vi "guerra.vi"(8 "carri difesa":i32, 11 "carri attacco":i32) -> (0 "difesa perde":bool, 2 "carri attacco\nrimanenti":i32, 3 "attacco perde":bool)   [LabVIEW 2013]
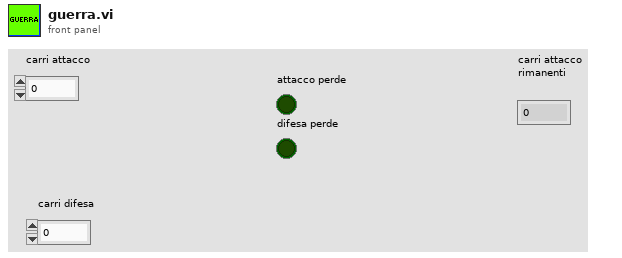
[diagram p1: front panel]
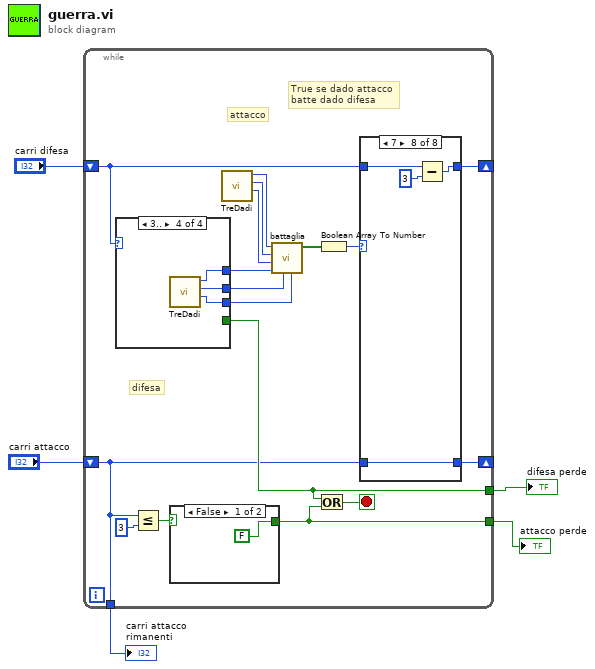
[diagram p0: block diagram]
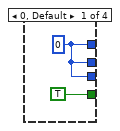
[diagram p2: hidden frame]
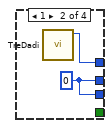
[diagram p3: hidden frame]
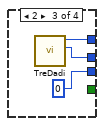
[diagram p4: hidden frame]
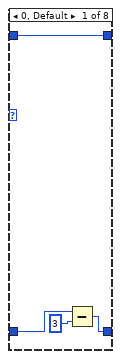
[diagram p5: hidden frame]
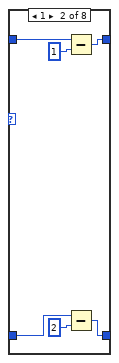
[diagram p6: hidden frame]
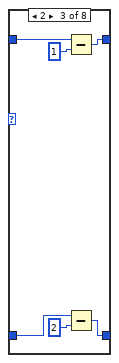
[diagram p7: hidden frame]
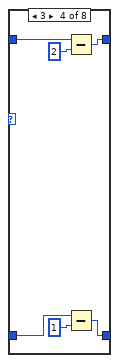
[diagram p8: hidden frame]
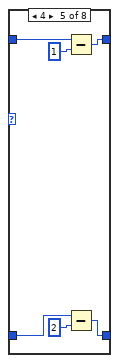
[diagram p9: hidden frame]
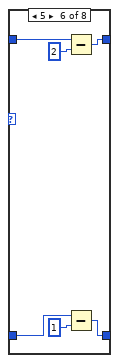
[diagram p10: hidden frame]
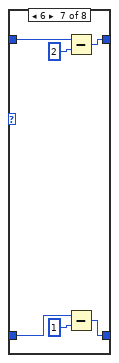
[diagram p11: hidden frame]
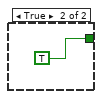
[diagram p12: hidden frame]
diagram:
  n1 = while {
    shift-right: [w11] -> _
    shift-left: "carri attacco" -> [w6]
    shift-right: [w10] -> _
    shift-left: "carri difesa" -> [w15]
    tunnel: [w7] -> w3
    tunnel: [w8] -> w2
    tunnel: [w6] -> w1
    stop <- w9 stop-if-true
    # "difesa"
    # "True se dado attacco\nbatte dado difesa"
    # "attacco"
    n2 = case shown="3.." w15 {
      tunnel: [w24 w26 w29 w32] -> w14
      tunnel: [w24 w25 w28 w31] -> w13
      tunnel: [w24 w25 u32 0 ("Dado_1") w30] -> w12
      tunnel: [TRUE _ _ _] -> w8
      frame 0, Default {
        w24 = u32 0 ("Dado_1")
      }
      frame 1 {
        w25 = 0
        n3 = call "TreDadi.vi"() -> ("Dado_1"=w26:u32)  [unwired: 9 in, 2 out]
      }
      frame 2 {
        n4 = call "TreDadi.vi"() -> ("Dado_2"=w28:u32, "Dado_1"=w29:u32)  [unwired: 9 in, 1 out]
      }
      frame 3.. {
        n5 = call "TreDadi.vi"() -> ("Dado_3"=w30:u32, "Dado_2"=w31:u32, "Dado_1"=w32:u32)  [unwired: 9 in]
      }
    }
    n6 = Less Or Equal?(x=w6, y=3) -> (x <= y?=w18:bool)
    n7 = case shown="False" w18 {
      tunnel: [FALSE TRUE] -> w7
      frame False {
      }
      frame True {
      }
    }
    n8 = call "TreDadi.vi"() -> ("Dado_3"=w20:u32, "Dado_2"=w21:u32, "Dado_1"=w22:u32)  [unwired: 9 in]
    n9 = call "battaglia.vi"("d3 difesa"=w12, "d2 difesa"=w13, "d1 difesa"=w14, "d3 attacco"=w20, "d2 attacco"=w21, "d1 attacco"=w22) -> ("risultati battaglia"=w17:bool[])  [unwired: 5 in]
    n10 = Or(x=w8, y=w7) -> (x .or. y?=w9:bool)
    n11 = Boolean Array To Number(Boolean array=w17) -> (number=w16:u32)
    n12 = case shown="7" w16 {
      tunnel: [w35 w41 w47 w53 w59 w65 w71 w74] -> w11
      tunnel: [w33 w39 w45 w51 w57 w63 w69 w75] -> w10
      tunnel: w6 -> [w34 w38 w44 w50 w56 w62 w68 w74]
      tunnel: w15 -> [w33 w37 w43 w49 w55 w61 w67 w73]
      frame 0, Default {
        n13 = Subtract(x=w34, y=3) -> (x-y=w35:i32)
      }
      frame 1 {
        n14 = Subtract(x=w37, y=1) -> (x-y=w39:i32)
        n15 = Subtract(x=w38, y=2) -> (x-y=w41:i32)
      }
      frame 2 {
        n16 = Subtract(x=w43, y=1) -> (x-y=w45:i32)
        n17 = Subtract(x=w44, y=2) -> (x-y=w47:i32)
      }
      frame 3 {
        n18 = Subtract(x=w49, y=2) -> (x-y=w51:i32)
        n19 = Subtract(x=w50, y=1) -> (x-y=w53:i32)
      }
      frame 4 {
        n20 = Subtract(x=w55, y=1) -> (x-y=w57:i32)
        n21 = Subtract(x=w56, y=2) -> (x-y=w59:i32)
      }
      frame 5 {
        n22 = Subtract(x=w61, y=2) -> (x-y=w63:i32)
        n23 = Subtract(x=w62, y=1) -> (x-y=w65:i32)
      }
      frame 6 {
        n24 = Subtract(x=w67, y=2) -> (x-y=w69:i32)
        n25 = Subtract(x=w68, y=1) -> (x-y=w71:i32)
      }
      frame 7 {
        n26 = Subtract(x=w73, y=3) -> (x-y=w75:i32)
      }
    }
  }
  "attacco perde" <- w3
  "difesa perde" <- w2
  "carri attacco\nrimanenti" <- w1
